vi "Logarithm Fit Coefficients (LAR).vi"(0 "Y":dbl[](array[numeric]), 5 "X":dbl[](array[numeric]), 7 "Weight":dbl[](array[numeric]), 9 "base of logarithm":dbl(ring)=2.71828 items=["e"=2.71828, "2"=2.0, "10"=10.0], 11 "tol":dbl=0.0001) -> (4 "amplitude":dbl, 6 "scale":dbl, 15 "error":i32)   [LabVIEW 2014, in "NI_AALPro.lvlib"]
uses:
  NI_AALPro.lvlib
  lvanlys.dll
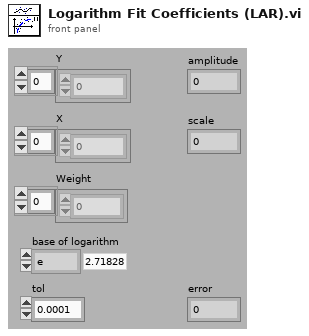
[diagram p1: front panel]
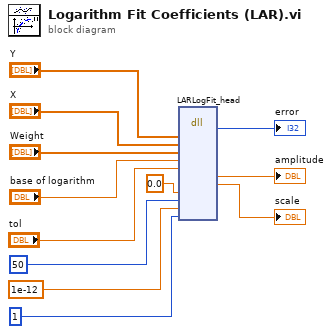
[diagram p0: block diagram]
diagram:
  n1 = dll-call lib="C:/Program Files (x86)/National Instruments/LabVIEW 2014/resource/lvanlys.*" fn="LARLogFit_head"("yH"="Y", "xH"="X", "weight"="Weight", "base"="base of logarithm", "tol"="tol", "meanErr"=0.0, "maxIter"=50, "absTol"=1e-12, "isCoef"=1) -> (→"error":i32, "amplitude"=→"amplitude":dbl, "scale"=→"scale":dbl)  [unwired: 14 in, 2 out]
